vi "dfd_Generalized Binomial Coefficients.vi"(8 "error in (no error)":errorcluster, 10 "k":i32, 11 "n":i32=1) -> (0 "error out":errorcluster, 3 "binomial coefficient (n,k)":dbl=1.0)   [LabVIEW 2017, in "NI_DigFilter_Process.lvlib"]
doc: "Calculates the binomial coefficient for integer values of <B>n</B> and <B>k</B>."
uses:
  <vilib>/addons/Digital Filter Design/NI_DigFilter_Process.lvlib
  <vilib>/addons/Digital Filter Design/_Misc.llb/dfd_Error Cluster From Error Code (Scalar).vi
  <vilib>/gmath/NI_Gmath.lvlib
  <vilib>/addons/Digital Filter Design/NI_DigFilterLicensed.lvlib
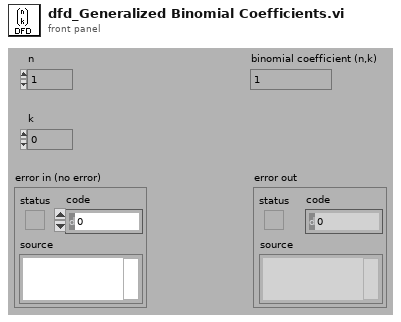
[diagram p1: front panel]
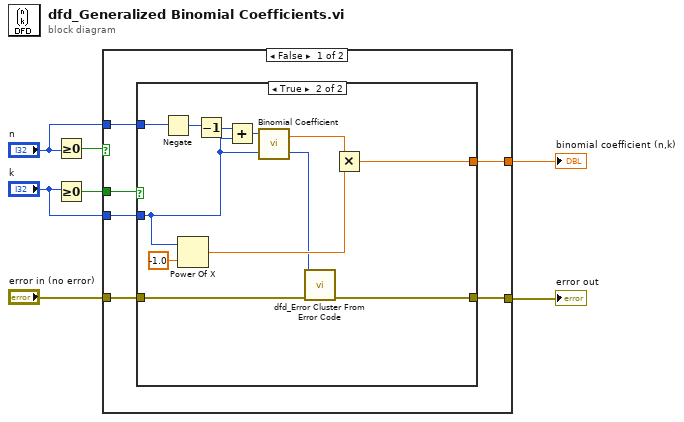
[diagram p0: block diagram]
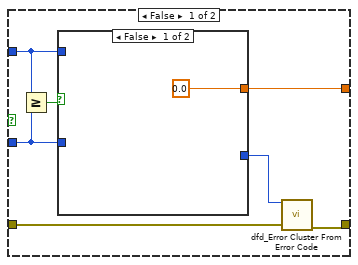
[diagram p2: hidden frame]
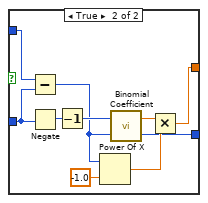
[diagram p3: hidden frame]
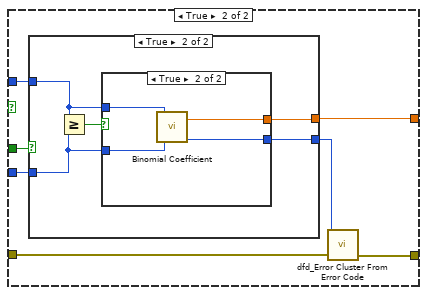
[diagram p4: hidden frame]
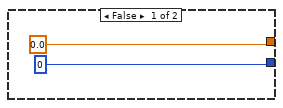
[diagram p5: hidden frame]
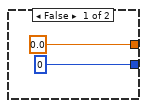
[diagram p6: hidden frame]
diagram:
  n1 = Greater Or Equal To 0?(x="n") -> (x >= 0?=w7:bool)
  n2 = Greater Or Equal To 0?(x="k") -> (x >= 0?=w6:bool)
  n3 = case shown="False" w7 {
    tunnel: w6 -> [w13 w50]
    tunnel: "n" -> [w11 w49]
    tunnel: "k" -> [w12 w48]
    tunnel: [w10 w47] -> w3
    tunnel: [w8 w45] -> w2
    tunnel: "error in (no error)" -> [w9 w44]
    frame False {
      n4 = case shown="True" w13 {
        tunnel: w12 -> [w18 w39]
        tunnel: w11 -> [w17 w42]
        tunnel: [w19 w35] -> w10
        tunnel: w9 -> [w16 w33]
        tunnel: [w15 w32] -> w8
        frame False {
          n5 = Greater Or Equal?(x=w17, y=w18) -> (x >= y?=w20:bool)
          n6 = case shown="False" w20 {
            tunnel: [0.0 w24] -> w19
            tunnel: w18 -> [_ w29]
            tunnel: w17 -> [_ w31]
            tunnel: [_ w22] -> w14
            frame False {
            }
            frame True {
              n7 = Subtract(x=w31, y=w29) -> (x-y=w26:i32)
              n8 = Negate(x=w29) -> (-x=w28:i32)
              n9 = Decrement(x=w28) -> (x-1=w27:i32)
              n10 = Power Of X(1:-1.0 ("x"), 2:w26) -> (0:w23:dbl)
              n11 = call <vilib>:"Binomial Coefficient.vi"("k"=w26, "n"=w27) -> ("error"=w22:i32, "binomial coefficient (n,k)"=w25:dbl)
              n12 = Multiply(x=w25, y=w23) -> (x*y=w24:dbl)
            }
          }
          n13 = call-poly <vilib>:"dfd_Error Cluster From Error Code.vi"("error in (no error)"=w16, "error code (0)"=w14) -> ("error out"=w15:errorcluster)  [unwired: 9 out]
        }
        frame True {
          n14 = Negate(x=w42) -> (-x=w41:i32)
          n15 = Power Of X(1:-1.0 ("x"), 2:w39) -> (0:w36:dbl)
          n16 = Decrement(x=w41) -> (x-1=w40:i32)
          n17 = Add(x=w40, y=w39) -> (x+y=w38:i32)
          n18 = call <vilib>:"Binomial Coefficient.vi"("k"=w39, "n"=w38) -> ("error"=w34:i32, "binomial coefficient (n,k)"=w37:dbl)
          n19 = call-poly <vilib>:"dfd_Error Cluster From Error Code.vi"("error in (no error)"=w33, "error code (0)"=w34) -> ("error out"=w32:errorcluster)  [unwired: 9 out]
          n20 = Multiply(x=w37, y=w36) -> (x*y=w35:dbl)
        }
      }
    }
    frame True {
      n21 = case shown="True" w50 {
        tunnel: w49 -> [_ w56]
        tunnel: w48 -> [_ w55]
        tunnel: [0 ("error") w54] -> w46
        tunnel: [0.0 ("binomial coefficient (n,k)") w53] -> w47
        frame False {
        }
        frame True {
          n22 = Greater Or Equal?(x=w56, y=w55) -> (x >= y?=w57:bool)
          n23 = case shown="True" w57 {
            tunnel: w56 -> [_ w63]
            tunnel: w55 -> [_ w62]
            tunnel: [0.0 ("binomial coefficient (n,k)") w61] -> w53
            tunnel: [0 ("error") w60] -> w54
            frame False {
            }
            frame True {
              n24 = call <vilib>:"Binomial Coefficient.vi"("k"=w62, "n"=w63) -> ("error"=w60:i32, "binomial coefficient (n,k)"=w61:dbl)
            }
          }
        }
      }
      n25 = call-poly <vilib>:"dfd_Error Cluster From Error Code.vi"("error in (no error)"=w44, "error code (0)"=w46) -> ("error out"=w45:errorcluster)  [unwired: 9 out]
    }
  }
  "binomial coefficient (n,k)" <- w3
  "error out" <- w2
